vi "Obtain Lock.vi"(8 "error in (no error)":errorcluster, 9 "timeout (-1 ms)":i32=-1 format="%d ms", 11 "Protected Pointer in":refnum<class "Protected Pointer.lvclass">) -> (0 "error out":errorcluster, 1 "timed out?":bool, 2 "lock status":bool, 3 "Protected Pointer out":refnum<class "Protected Pointer.lvclass">)   [LabVIEW 2016, in "Memory Manager.lvlib" / "Protected Pointer.lvclass"]
uses:
  Protected Pointer.lvclass
  Invalid Lock.vi
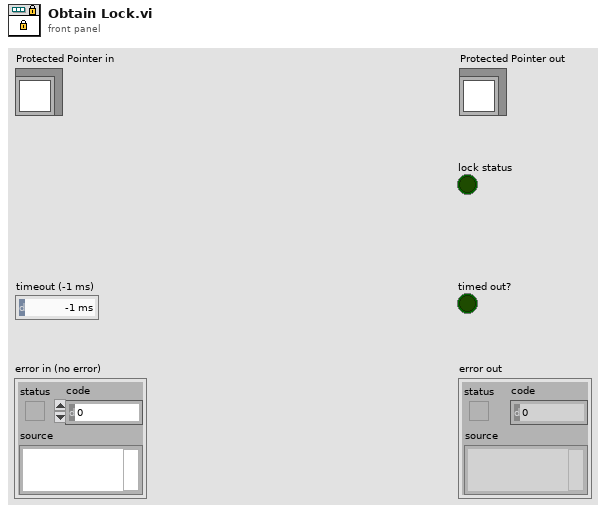
[diagram p1: front panel]
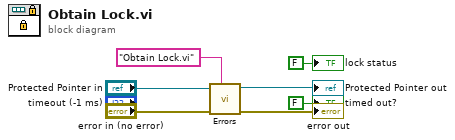
[diagram p0: block diagram]
diagram:
  n1 = call-poly "Errors.vi"("source vi name"="Obtain Lock.vi", "error in (no error)"="error in (no error)", "Lockable Pointer in"="Protected Pointer in") -> ("error out"=→"error out":errorcluster, "Lockable Pointer out"=→"Protected Pointer out":refnum<class "Protected Pointer.lvclass">)  [unwired: 7 in]
  "timed out?" <- FALSE ("timed out?")
  "lock status" <- FALSE ("lock status")
